vi "DisplayManager_test.vi"() -> ()   [LabVIEW 2014]
uses:
  DataTypes/DataTypes.llb/Indexes.ctl
panel:
  out "BWCrop":T1(plugin-control)
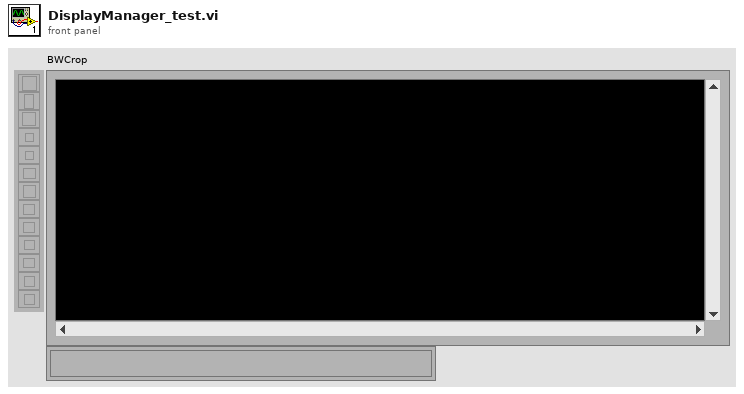
[diagram p1: front panel]
types:
  T1 = typedef "IMAQ Image.ctl" = refnum<image>
  T2 = typedef "Indexes.ctl" = cluster{"BASE COLOR":dbl[], "COLOR1":dbl[], "COLOR2":dbl[], "COLOR3":dbl[], "COLOR4":dbl[], "COLOR5":dbl[]}
  T3 = typedef "RTG.ctl" = cluster{"Radiogram":T1, "Thresholded":T1, "Weld":T1, "Labeled":T1}
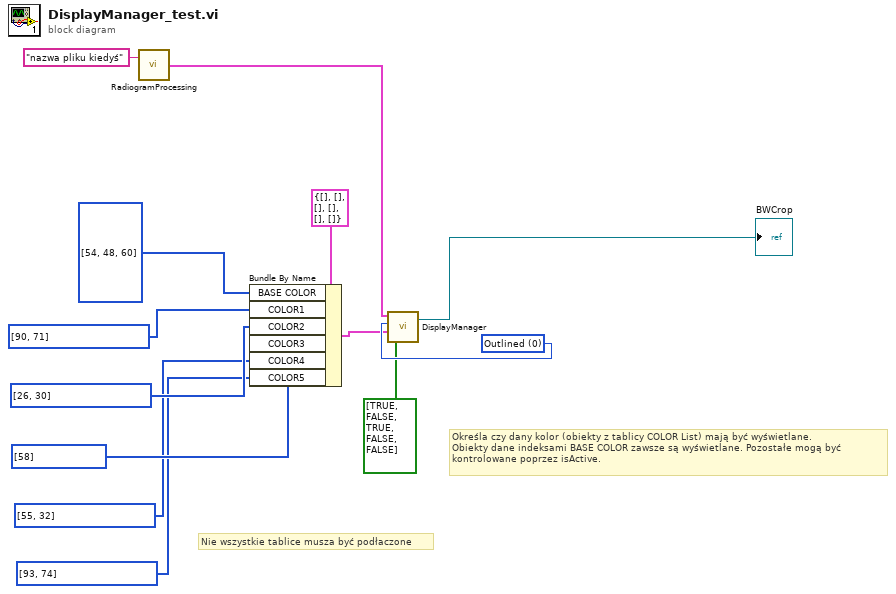
[diagram p0: block diagram]
diagram:
  w11 = u8 0 items=["Outlined", "Filled", ""] ("Display type")
  # "Określa czy dany kolor (obiekty z tablicy COLOR List) mają być wyświetlane.\nObiekty dane indeksami BASE COLOR zawsze są wyświetlane. Pozostałe mogą być \nkontrolowane poprzez isActive."
  # "Nie wszystkie tablice musza być podłaczone"
  n1 = call "RadiogramProcessing.vi"("FileName"="nazwa pliku kiedyś") -> ("RTGDataPack"=w2:T3)  [unwired: 1 in]
  n2 = Bundle By Name(cluster=T2 {"BASE COLOR"=[], "COLOR1"=[], "COLOR2"=[], "COLOR3"=[], "COLOR4"=[], "COLOR5"=[]} ("Color Indexes"), "BASE COLOR"=u32[] [54, 48, 60] ("Labels In"), "COLOR1"=u32[] [90, 71], "COLOR2"=u32[] [26, 30], "COLOR3"=i32[] [58], "COLOR4"=u32[] [55, 32], "COLOR5"=u32[] [93, 74]) -> (w3:T2)
  n3 = call "DisplayManager.vi"("isColorActive"=bool[] [TRUE, FALSE, TRUE, FALSE, FALSE], "Color Lists"=w3, "Display type"=w11, "RTGDataPack"=w2) -> ("Output Image"=→"BWCrop":T1)  [unwired: 1 in]
